vi "GEOM_Line2Overrwcs2.vi"(9 "curr arr":string[][](array[string]), 10 "extension data":string) -> (2 "out":string[][](array[string]))   [LabVIEW 2016]
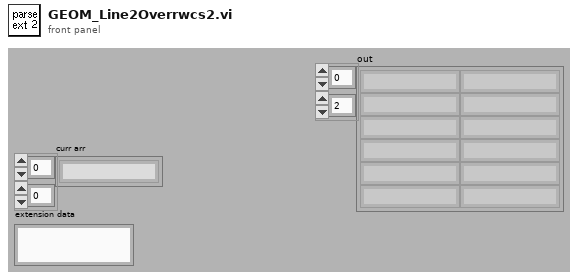
[diagram p1: front panel]
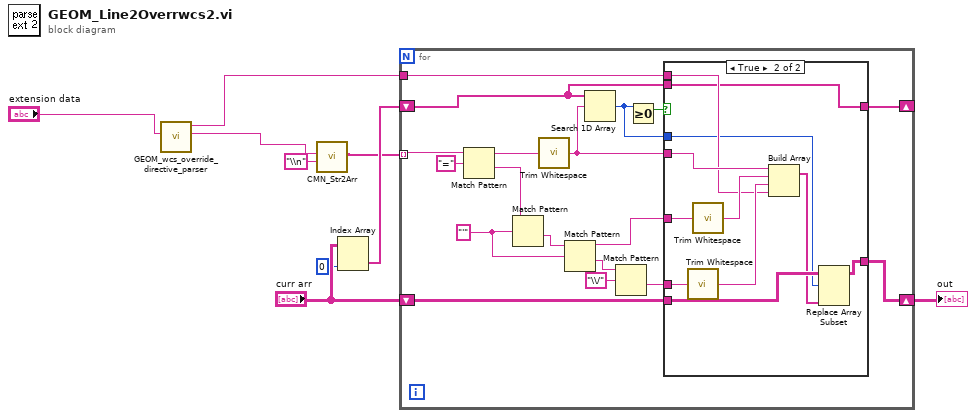
[diagram p0: block diagram]
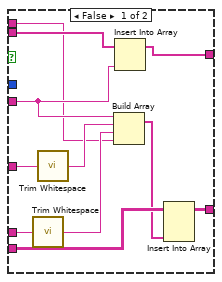
[diagram p2: hidden frame]
diagram:
  n1 = call "GEOM_wcs_override_directive_parser.vi"("modif in"="extension data") -> ("modif out"=w1:string, "last col"=w2:string)  [unwired: 9 out]
  n2 = call "CMN_Str2Arr.vi"("separator"="\\n", "string in"=w1) -> ("Array out"=w4:string[])  [unwired: 2 in, 7 out]
  n3 = Index Array(array="curr arr", index (col)=0 ("disabled index (col)")) -> (element=w6:string[])  [unwired: 1 in]
  n4 = for {
    tunnel: w4 -> [w27] mode=indexing
    shift-right: [w18] -> w9
    shift-left: "curr arr" -> [w19]
    shift-right: [w15] -> _
    shift-left: w6 -> [w17]
    tunnel: w2 -> [w10]
    w23 = "'" ("regular expression")
    n5 = Match Pattern(string=w27, regular expression="=") -> (before substring=w25:string, after substring=w24:string)  [unwired: 3 out]
    n6 = Match Pattern(string=w24, regular expression=w23) -> (after substring=w21:string)  [unwired: 4 out]
    n7 = call <vilib>:"Trim Whitespace.vi"("string"=w25) -> ("trimmed string"=w16:string)  [unwired: 1 in]
    n8 = Match Pattern(string=w21, regular expression=w23) -> (before substring=w22:string, after substring=w13:string)  [unwired: 3 out]
    n9 = Search 1D Array(1D array=w17, element=w16) -> (index of element=w14:i32)  [unwired: 1 out]
    n10 = Match Pattern(string=w13, regular expression="\\/") -> (after substring=w11:string)  [unwired: 4 out]
    n11 = Greater Or Equal To 0?(x=w14) -> (x >= 0?=w20:bool)
    n12 = case shown="True" w20 {
      tunnel: w22 -> [w37 w48]
      tunnel: w16 -> [w32 w45]
      tunnel: w19 -> [w36 w47]
      tunnel: [w34 w46] -> w18
      tunnel: w17 -> [w33 w39]
      tunnel: [w31 w39] -> w15
      tunnel: w14 -> [_ w41]
      tunnel: w11 -> [w30 w44]
      tunnel: w10 -> [w28 w42]
      frame False {
        n13 = call <vilib>:"Trim Whitespace.vi"("string"=w30) -> ("trimmed string"=w29:string)  [unwired: 1 in]
        n14 = call <vilib>:"Trim Whitespace.vi"("string"=w37) -> ("trimmed string"=w38:string)  [unwired: 1 in]
        n15 = Build Array(w32, w38, w29, w28) -> (w35:string[])
        n16 = Insert Into Array(array=w33, new element=w32) -> (w31:string[])  [unwired: 1 in]
        n17 = Insert Into Array(array=w36, new element=w35) -> (w34:string[][])  [unwired: 2 in]
      }
      frame True {
        n18 = call <vilib>:"Trim Whitespace.vi"("string"=w44) -> ("trimmed string"=w43:string)  [unwired: 1 in]
        n19 = call <vilib>:"Trim Whitespace.vi"("string"=w48) -> ("trimmed string"=w49:string)  [unwired: 1 in]
        n20 = Build Array(w45, w49, w43, w42) -> (w40:string[])
        n21 = Replace Array Subset(array=w47, new element=w40, index (row)=w41) -> (w46:string[][])  [unwired: 1 in]
      }
    }
  }
  "out" <- w9
